vi "Get Sweep.vi"(0 "Vector Path in":refnum<class "Vector Path.lvclass">, 5 "Sweep Name":string, 11 "error in (no error)":errorcluster) -> (4 "Vector Path out":refnum<class "Vector Path.lvclass">, 6 "Sweep":T1, 8 "Sweep not found?":bool, 15 "error out":errorcluster)   [LabVIEW 2023, in "RFFixtureCharact.Public.lvlib" / "Vector Path.lvclass"]
uses:
  Public/Base Classes/Vector/Vector Path Group/Type Definitions/Sweep.ctl
  Public/Base Classes/Vector/Vector Path/Vector Path.lvclass
  Public/Base Classes/Vector/Vector Path/Vector Path.lvclass/Vector Path.ctl
  Common/RFCalAndFixtureCharact.Common.lvlib
  Public/Base Classes/Vector/Vector Path Group/Vector Path Group.lvclass
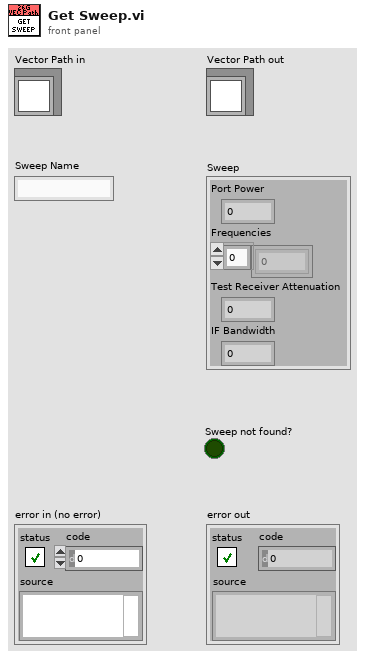
[diagram p1: front panel]
types:
  T1 = typedef "RFFixtureCharact.Public.lvlib/Vector Path Group.lvclass/Sweep.ctl" = cluster{"Port Power":dbl, "Frequencies":dbl[], "Test Receiver Attenuation":dbl, "IF Bandwidth":dbl}
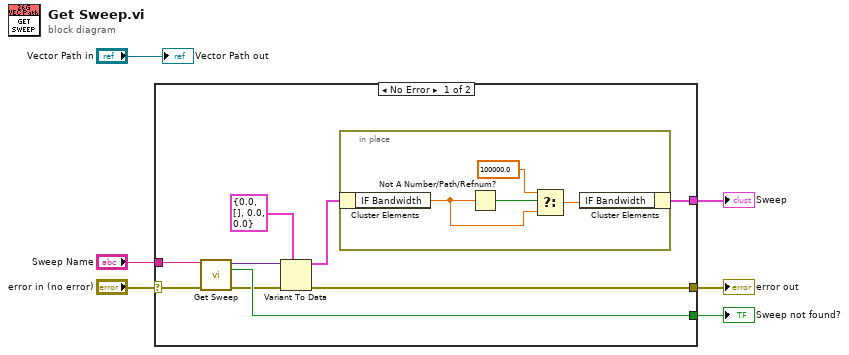
[diagram p0: block diagram]
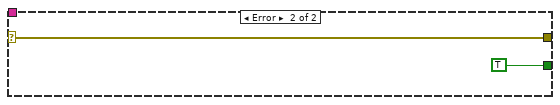
[diagram p2: hidden frame]
diagram:
  n1 = case shown="No Error" "error in (no error)" {
    selector: "error in (no error)" -> [w11 w21]
    tunnel: "Sweep Name" -> [w15 _]
    tunnel: [w9 w21] -> w5
    tunnel: [w14 TRUE ("Sweep not found?")] -> w4
    tunnel: [w7 _] -> w3
    frame No Error {
      n2 = call "Get Sweep.vi"("Sweep Name"=w15, "error in (no error)"=w11) -> ("Variant"=w12:variant, "Sweep not found?"=w14:bool, "error out"=w10:errorcluster)  [unwired: 11 in]
      n3 = Variant To Data(error in=w10, type=T1 {"Port Power"=0.0, "Frequencies"=[], "Test Receiver Attenuation"=0.0, "IF Bandwidth"=0.0} ("Sweep"), Variant=w12) -> (data=w8:T1, error out=w9:errorcluster)
      n4 = in-place {
        n5 = in-place-cluster #1(w8) -> ("IF Bandwidth"=w17:dbl)
        n6 = Not A Number/Path/Refnum?(number/path/refnum=w17) -> (NaN/Path/Refnum?=w16:bool)
        n7 = Select(t=100000.0, s=w16, f=w17) -> (s? t:f=w18:dbl)
        n8 = in-place-cluster #1("IF Bandwidth"=w18) -> (w7:T1)
      }
    }
    frame Error {
    }
  }
  "error out" <- w5
  "Sweep not found?" <- w4
  "Sweep" <- w3
  "Vector Path out" <- "Vector Path in"
